vi "SampleErrorUXFile.vi"(8 "error in (no error)":errorcluster) -> (0 "error out":errorcluster)   [LabVIEW 2019, in "LabErrorUX.lvclass"]
uses:
  LabErrorUX.lvclass
  <vilib>/SLL Toolkit/SLL File IO/Spreadsheet/SLL Spreadsheet.lvlib
panel:
  in  "File Path":path=path "D:/Github/KarthikAbiram/LabErrorUX/Source/SampleLabErrorUX.csv"
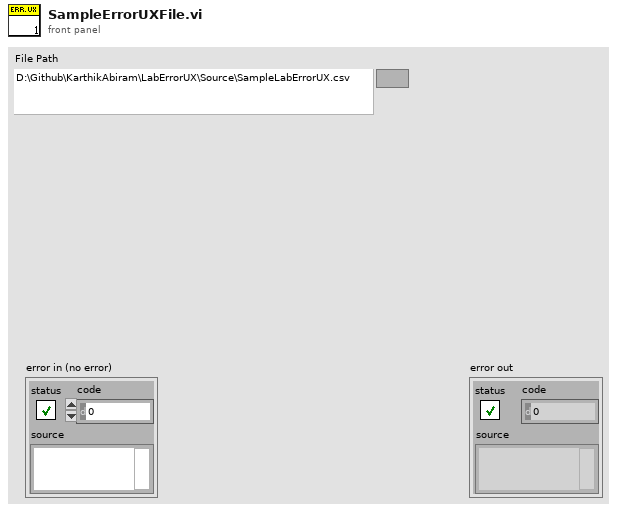
[diagram p1: front panel]
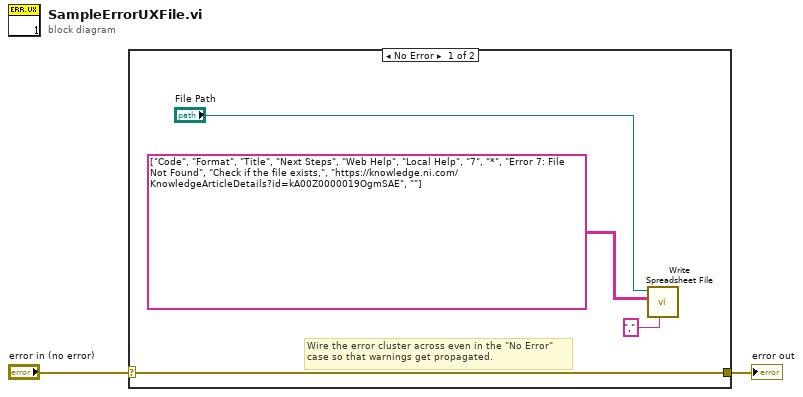
[diagram p0: block diagram]
diagram:
  n1 = case shown="No Error" "error in (no error)" {
    selector: "error in (no error)" -> [w6 w7]
    tunnel: [w6 w7] -> w1
    frame No Error {
      # "Wire the error cluster across even in the \"No Error\"\ncase so that warnings get propagated."
      n2 = call <vilib>:"Write Spreadsheet File.vi"("Delimiter (tab)"=",", "2D String[][]"=string[][] [["Code", "Format", "Title", "Next Steps", "Web Help", "Local Help"], ["7", "*", "Error 7: File Not Found", "Check if the file exists,", "https://knowledge.ni.com/KnowledgeArticleDetails?id=kA00Z0000019OgmSAE", ""]], "File Path"="File Path") -> ()  [unwired: 7 in, 2 out]
    }
    frame Error {
    }
  }
  "error out" <- w1
